vi "Configure Arbitrary Waveform.vi"(7 "Number of Waveforms (1)":dbl=1.0, 8 "error in (no error)":errorcluster, 9 "Shape of Waveform (3: Square)":i32(ring)=3 items=["Exponential", "Ramp", "Sinusoid", "Square", "Trapezoid", "Triangle", "User Defined"], 10 "Output Channel (0: Channel 1)":i32(ring) items=["Channel 1", "Channel 2"], 11 "VISA resource name":refnum<visa-resource-name>) -> (0 "error out":errorcluster, 3 "VISA resource name out":refnum<visa-resource-name>)   [LabVIEW 2023, in "Agilent B2900 Series.lvlib"]
doc: "Configure the arbitrary waveform output.\n\n<B>Note:</B>\nThis VI is only supported by Agilent models B2961A, B2962A, B2961B,B2962B,B2961C and B2962C"
uses:
  Agilent B2900 Series.lvlib
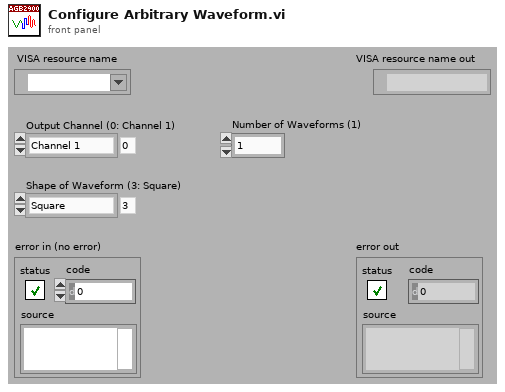
[diagram p1: front panel]
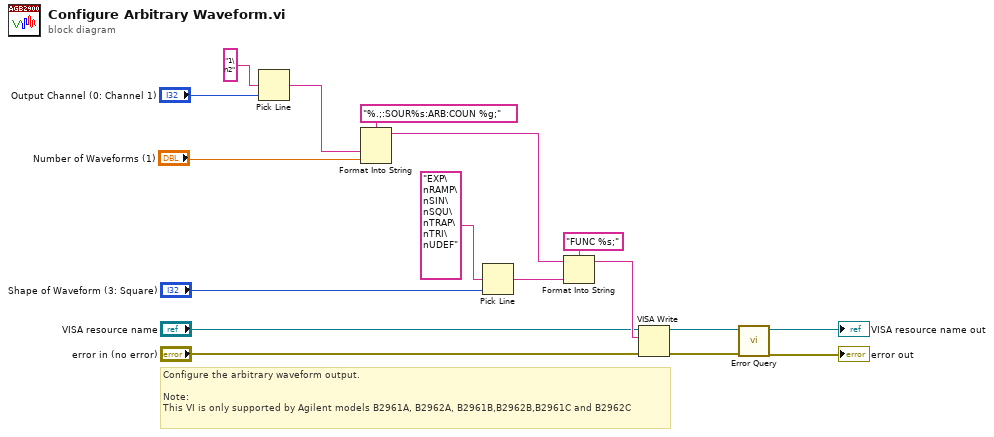
[diagram p0: block diagram]
diagram:
  # "Configure the arbitrary waveform output.\n\nNote:\nThis VI is only supported by Agilent models B2961A, B2962A, B2961B,B2962B,B2961C and B2962C"
  n1 = Pick Line(multi-line string="1\n2" ("string (\"\")"), line index="Output Channel (0: Channel 1)") -> (output string=w5:string)  [unwired: 1 in]
  n2 = Format Into String(format string="%.;:SOUR%s:ARB:COUN %g;", w5, "Number of Waveforms (1)") -> (resulting string=w1:string)  [unwired: 2 in, 1 out]
  n3 = Pick Line(multi-line string="EXP\nRAMP\nSIN\nSQU\nTRAP\nTRI\nUDEF" ("string (\"\")"), line index="Shape of Waveform (3: Square)") -> (output string=w2:string)  [unwired: 1 in]
  n4 = Format Into String(format string="FUNC %s;", initial string=w1, w2) -> (resulting string=w15:string)  [unwired: 1 in, 1 out]
  n5 = VISA Write(VISA resource name="VISA resource name", write buffer=w15, error in (no error)="error in (no error)") -> (VISA resource name out=w12:refnum<visa-resource-name>, error out=w11:errorcluster)  [unwired: 1 out]
  n6 = call "Error Query.vi"("error in (no error)"=w11, "VISA resource name"=w12) -> ("error out"=→"error out":errorcluster, "VISA resource name out"=→"VISA resource name out":refnum<visa-resource-name>)  [unwired: 8 out]
